vi "Read Port.vi"(0 "NXP in":refnum<class "NXP.lvclass">, 5 "VISA resource name":refnum<visa-resource-name>, 7 "Port":dbl, 11 "error in (no error)":errorcluster) -> (4 "NXP out":refnum<class "NXP.lvclass">, 6 "VISA resource name 2":refnum<visa-resource-name>, 8 "Binary Number":T1, 10 "Response":string, 15 "error out":errorcluster)   [LabVIEW 2020, in "NXP.lvclass"]
uses:
  NXP.lvclass
  aae82f05-5fd1-4f52-aee5-bd24a4559ed3.vi
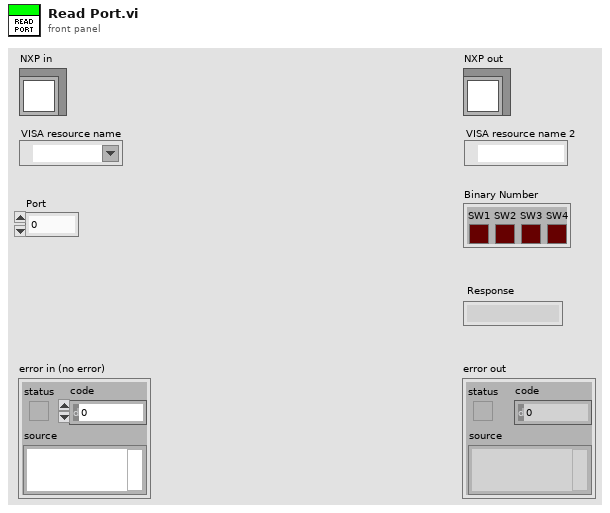
[diagram p1: front panel]
types:
  T1 = cluster{"SW1":bool, "SW2":bool, "SW3":bool, "SW4":bool, "[4]":bool, "[5]":bool, "[6]":bool, "[7]":bool, "[8]":bool}
  T2 = enum16{"Write", "Read", "Config", "Reset", "Close"}
  T3 = cluster{"[0]":bool, "[1]":bool, "[2]":bool, "[3]":bool, "[4]":bool, "[5]":bool, "[6]":bool, "[7]":bool, "[8]":bool}
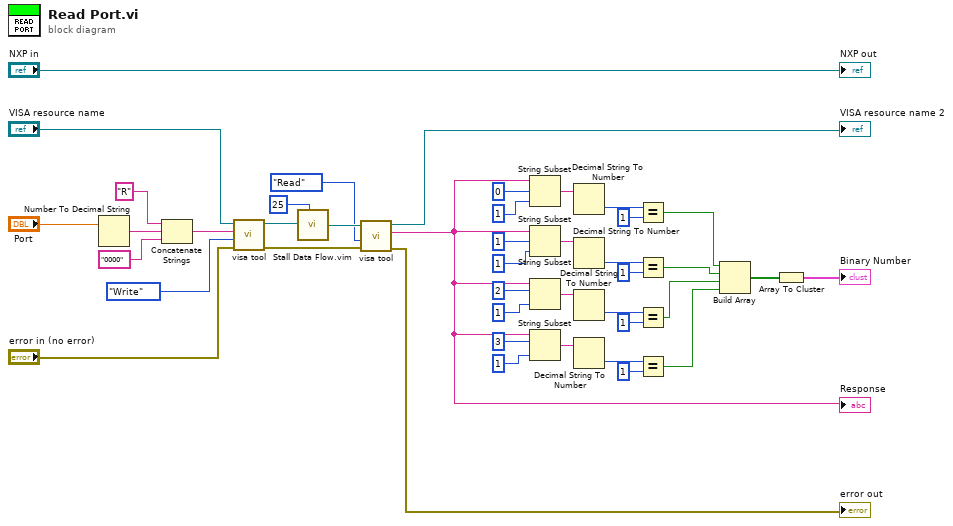
[diagram p0: block diagram]
diagram:
  n1 = Number To Decimal String(number="Port") -> (decimal integer string=w4:string)  [unwired: 1 in]
  n2 = Concatenate Strings("R" ("string"), w4, "0000" ("string")) -> (w3:string)
  n3 = call "visa tool.vi"("error in (no error)"="error in (no error)", "Opciones"=T2."Write", "Write"=w3, "VISA com port"="VISA resource name") -> ("error out"=w37:errorcluster, "VISA com port 2"=w41:refnum<visa-resource-name>)  [unwired: 5 in, 1 out]
  n4 = call "Stall Data Flow.vim"("value in"=w41, "milliseconds to wait"=u32 25) -> ("value out"=w40:refnum<visa-resource-name>)  [unwired: 1 out]
  n5 = call "visa tool.vi"("error in (no error)"=w37, "Opciones"=T2."Read", "VISA com port"=w40) -> ("error out"=→"error out":errorcluster, "Read"=w11:string, "VISA com port 2"=→"VISA resource name 2":refnum<visa-resource-name>)  [unwired: 6 in]
  "Response" <- w11
  n6 = String Subset(string=w11, offset (0)=0, length (rest)=1 ("length (rest)")) -> (substring=w28:string)
  n7 = String Subset(string=w11, offset (0)=1, length (rest)=1 ("length (rest)")) -> (substring=w27:string)
  n8 = String Subset(string=w11, offset (0)=2, length (rest)=1 ("length (rest)")) -> (substring=w26:string)
  n9 = String Subset(string=w11, offset (0)=3, length (rest)=1 ("length (rest)")) -> (substring=w25:string)
  n10 = Decimal String To Number(string=w28) -> (number=w24:i32)  [unwired: 2 in, 1 out]
  n11 = Decimal String To Number(string=w27) -> (number=w19:i32)  [unwired: 2 in, 1 out]
  n12 = Decimal String To Number(string=w26) -> (number=w18:i32)  [unwired: 2 in, 1 out]
  n13 = Decimal String To Number(string=w25) -> (number=w17:i32)  [unwired: 2 in, 1 out]
  n14 = Equal?(x=w24, y=1) -> (x = y?=w16:bool)
  n15 = Equal?(x=w19, y=1) -> (x = y?=w15:bool)
  n16 = Equal?(x=w18, y=1) -> (x = y?=w14:bool)
  n17 = Equal?(x=w17, y=1) -> (x = y?=w13:bool)
  n18 = Build Array(w16, w15, w14, w13) -> (w12:bool[])
  n19 = Array To Cluster(array=w12) -> (cluster=→"Binary Number":T3)
  "NXP out" <- "NXP in"
